vi "ScanAction.vi"(8 "error in (no error)":errorcluster caption="entrée d'erreur (pas d'erreur)", 9 "IndicePoint":i32, 11 "LSCI332 In":refnum<class "LSCI332.lvclass"> caption="DNL_LabVIEW Object in") -> (0 "error out":errorcluster caption="sortie d'erreur", 2 "ScanParsOut":dbl[](array[numeric]), 3 "LSCI332 Out":refnum<class "LSCI332.lvclass"> caption="DNL_LabVIEW Object out")   [LabVIEW 2012, in "LSCI332.lvclass"]
uses:
  LSCI332.lvclass
  LSCI332.lvclass/LSCI332.ctl
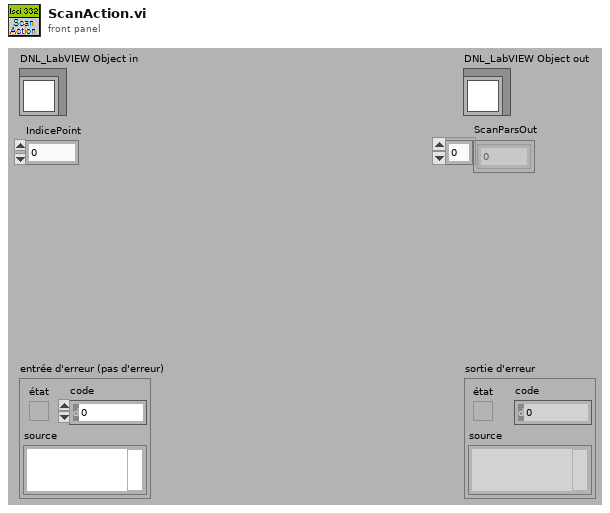
[diagram p1: front panel]
types:
  T1 = typedef "LSCI332.lvclass/LSCI332_Func.ctl" = enum16{"Read_InputA (K,S)", "Read_InputA&Heater (K,S,%,W)", "Read_InputB (K,S)", "Read_InputB&Heater (K,S,%,W)", "Read_Heater (%,W)", "Read_InputA&B(K,S,K,S)", "Read_InputA&B&Heater (K,S,K,S,%,W)", "Scan_Loop1(K,S)", "Scan_Loop2(K,S)"}
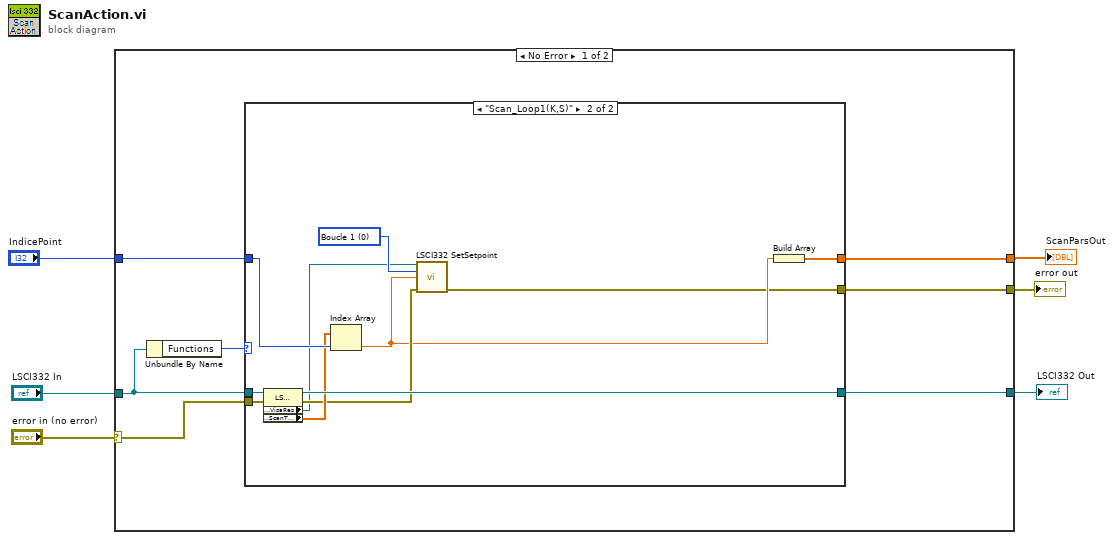
[diagram p0: block diagram]
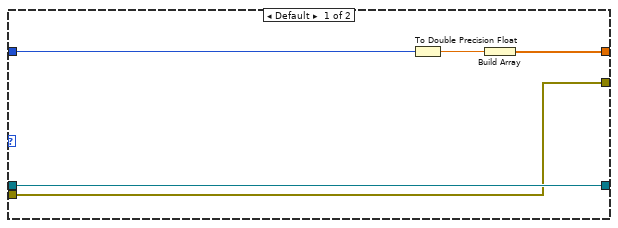
[diagram p2: hidden frame]
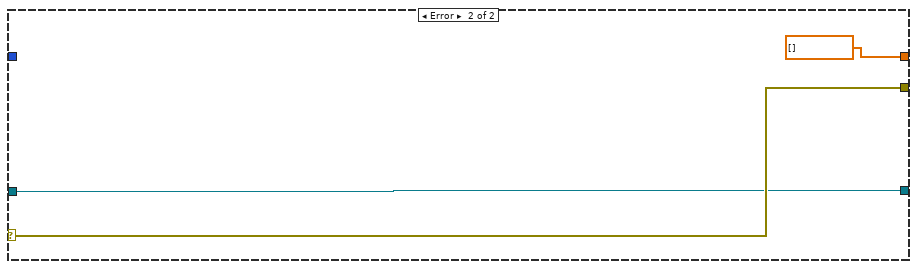
[diagram p3: hidden frame]
diagram:
  n1 = case shown="No Error" "error in (no error)" {
    selector: "error in (no error)" -> [w10 w32]
    tunnel: "LSCI332 In" -> [w11 w31]
    tunnel: [w9 dbl[] []] -> w1
    tunnel: [w8 w32] -> w4
    tunnel: [w7 w31] -> w3
    tunnel: "IndicePoint" -> [w12 _]
    frame No Error {
      n2 = Unbundle By Name(w11) -> ("Functions"=w13:T1)
      n3 = case shown="\"Scan_Loop1(K,S)\"" w13 {
        tunnel: [w14 w22] -> w9
        tunnel: w12 -> [w18 w25]
        tunnel: [w16 w27] -> w7
        tunnel: w11 -> [w16 w29]
        tunnel: w10 -> [w15 w28]
        tunnel: [w15 w19] -> w8
        frame Default {
          n4 = To Double Precision Float(number=w18) -> (double precision float=w17:dbl)
          n5 = Build Array(w17) -> (w14:dbl[])
        }
        frame "Scan_Loop1(K,S)" {
          w26 = u32 0 items=["Boucle 1", "Boucle 2"] ("Boucle(1)")
          n6 = property class="LSCI332.lvclass"(reference=w29, error in=w28) -> (reference out=w27:refnum<class "LSCI332.lvclass">, error out=w23:errorcluster, "Accessor:VisaRes"=w20:refnum<visa-resource-name>, "Accessor:ScanTable"=w24:dbl[])
          n7 = Index Array(array=w24, index=w25) -> (element=w21:dbl)
          n8 = call <userlib>:"LSCI332 SetSetpoint.vi"("VISA Rsrc"=w20, "Boucle(1)"=w26, "SetPoint"=w21, "error in (no error)"=w23) -> ("error out"=w19:errorcluster)  [unwired: 11 in]
          n9 = Build Array(w21) -> (w22:dbl[])
        }
      }
    }
    frame Error {
    }
  }
  "error out" <- w4
  "LSCI332 Out" <- w3
  "ScanParsOut" <- w1
